vi "Transform And Project.vi"(11 "Core Data":T1={"Screen Dimensions"={"Width"=0, "Height"=0}, "Camera"={"Field Of View"=0.0, "Near Plane"=0.0, "Far Plane"=0.0}, "Transform"={"Position"={"x"=0.0, "y"=0.0, "z"=0.0}, "Rotation"={"x"=0.0, "y"=0.0, "z"=0.0}, "Scale"={"x"=0.0, "y"=0.0, "z"=0.0}}, "Line Colour"=0, "Fill Colour"=0, "Draw Lines"=FALSE, "Projection Matrix"=[], "Update Screen"=FALSE, "Frame Buffer"=refnum, "Objects"=[], "Camera Up"=2.6797385, "Camera Left"=2.6797385, "Camera Rotation"=2.6797385, "Camera Forward"=2.6797385, "Draw Triangles"=FALSE, "Frame Buffer 2"=refnum, "Framebuffer"=FALSE} {"Camera Forward" scale=-10.0..10.0; "Camera Rotation" scale=-90.0..90.0; "Camera Left" scale=-10.0..10.0; "Camera Up" scale=-10.0..10.0}) -> (2 "Delta Time [s]":dbl format="%.3p", 3 "Triangles Sorted":T8[](array[typedef]))   [LabVIEW 2022 SP3]
uses:
  Libraries/3D/Triangle 2D.ctl
  Libraries/3D/Point 2D.ctl
  Core Data.ctl
  Libraries/Raster/Screen Dimensions.ctl
  Libraries/3D/Camera.ctl
  Libraries/3D/Transform.ctl
  Libraries/3D/Vector 3D.ctl
  Libraries/3D/Mesh.ctl
  Libraries/3D/Triangle 3D.ctl
  <vilib>/Utility/High Resolution Relative Seconds.vi
  Libraries/3D/3D.lvlib
  Libraries/Utility/Utility.lvlib
  Libraries/Raster/Raster.lvlib
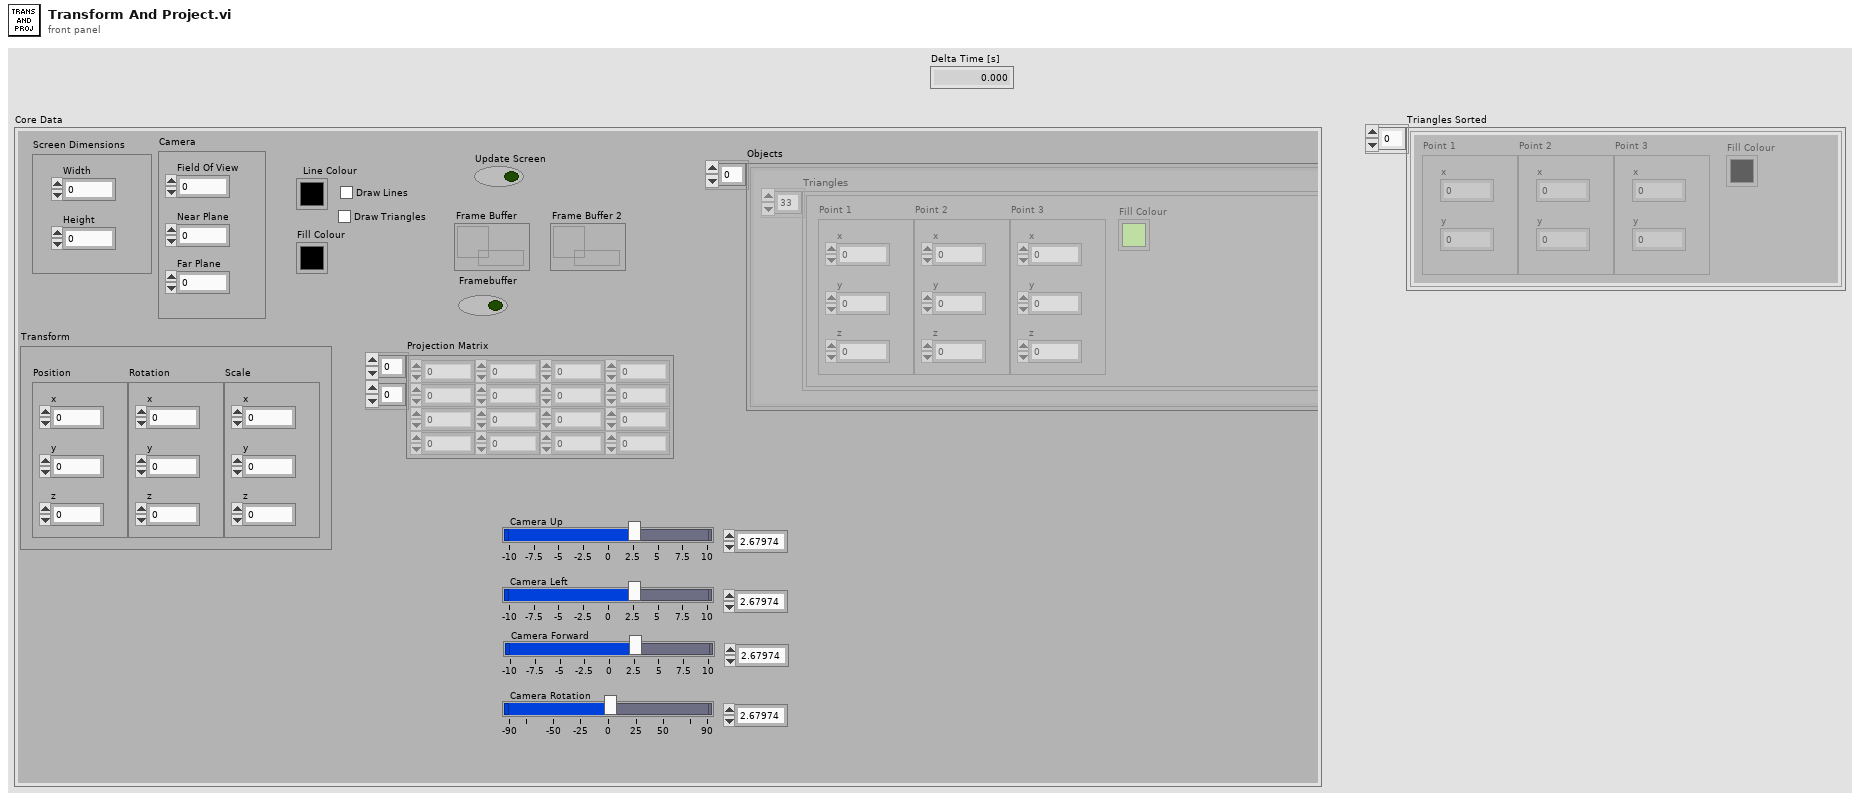
[diagram p1: front panel]
types:
  T1 = typedef "Core Data.ctl" = cluster{"Screen Dimensions":T2, "Camera":T3, "Transform":T4, "Line Colour":u32, "Fill Colour":u32, "Draw Lines":bool, "Projection Matrix":sgl[][], "Update Screen":bool, "Frame Buffer":refnum<data-value>, "Objects":T6[], "Camera Up":sgl, "Camera Left":sgl, "Camera Rotation":sgl, "Camera Forward":sgl, "Draw Triangles":bool, "Frame Buffer 2":refnum<data-value>, "Framebuffer":bool}
  T2 = typedef "Raster.lvlib/Screen Dimensions.ctl" = cluster{"Width":u32, "Height":u32}
  T3 = typedef "3D.lvlib/Camera.ctl" = cluster{"Field Of View":sgl, "Near Plane":sgl, "Far Plane":sgl}
  T4 = typedef "3D.lvlib/Transform.ctl" = cluster{"Position":T5, "Rotation":T5, "Scale":T5}
  T5 = typedef "3D.lvlib/Vector 3D.ctl" = cluster{"x":sgl, "y":sgl, "z":sgl}
  T6 = typedef "3D.lvlib/Mesh.ctl" = cluster{"Triangles":T7[]}
  T7 = typedef "3D.lvlib/Triangle 3D.ctl" = cluster{"Point 1":T5, "Point 2":T5, "Point 3":T5, "Fill Colour":u32}
  T8 = typedef "3D.lvlib/Triangle 2D.ctl" = cluster{"Point 1":T9, "Point 2":T9, "Point 3":T9, "Fill Colour":u32}
  T9 = typedef "3D.lvlib/Point 2D.ctl" = cluster{"x":sgl, "y":sgl}
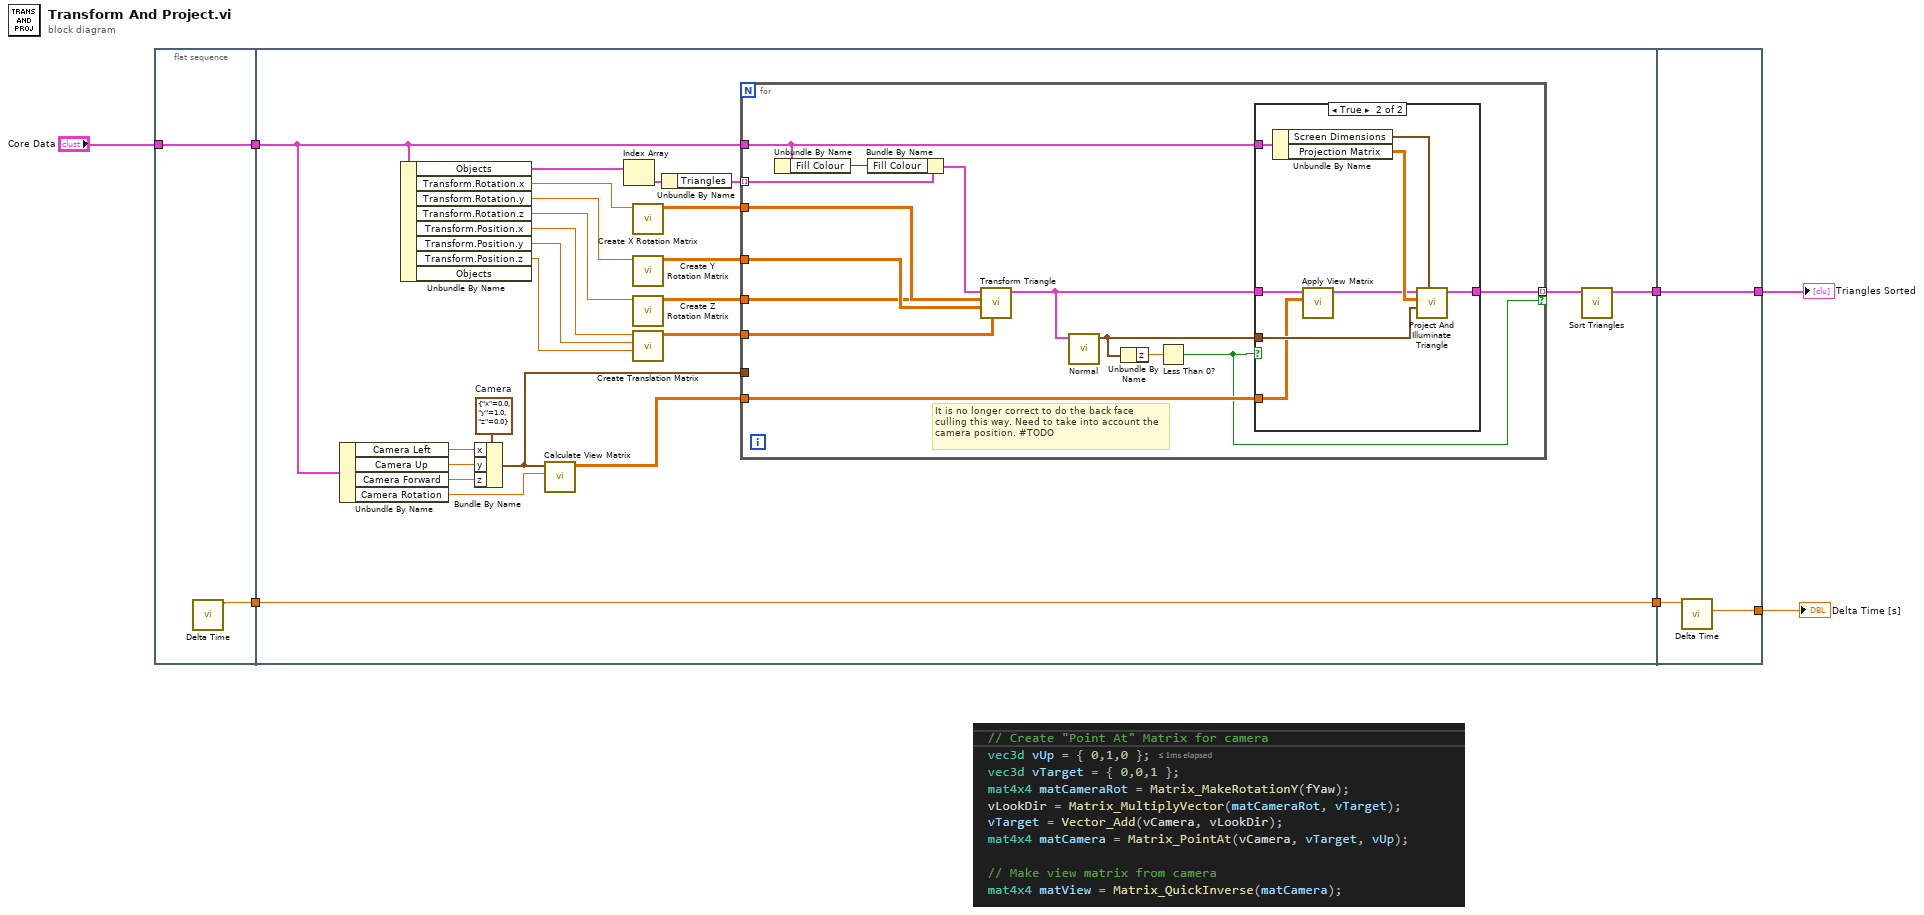
[diagram p0: block diagram]
diagram:
  n1 = flat-sequence {
    tunnel: "Core Data" -> [w9]
    tunnel: [w9] -> w3
    tunnel: [w8] -> w1
    tunnel: [w33] -> w5
    tunnel: w3 -> [w18]
    tunnel: [w10] -> w2
    tunnel: w1 -> [w10]
    tunnel: [w58] -> w7
    tunnel: w5 -> [w58]
    tunnel: [w57] -> w4
    tunnel: w2 -> [w56]
    frame #0 {
      n2 = call "Delta Time.vi"() -> ("Relative Seconds Out"=w8:dbl)  [unwired: 10 in, 1 out]
    }
    frame #1 {
      w17 = T5 {"x"=0.0, "y"=1.0, "z"=0.0}  # Camera
      n3 = Unbundle By Name(w18) -> ("Camera Left"=w12:sgl, "Camera Up"=w13:sgl, "Camera Forward"=w16:sgl, "Camera Rotation"=w14:sgl)
      n4 = Unbundle By Name(w18) -> ("Objects"=w32:T6[], "Transform.Rotation.x"=w26:sgl, "Transform.Rotation.y"=w27:sgl, "Transform.Rotation.z"=w28:sgl, "Transform.Position.x"=w20:sgl, "Transform.Position.y"=w19:sgl, "Transform.Position.z"=w29:sgl)  [unwired: 1 out]
      n5 = Bundle By Name(cluster=w17, "x"=w12, "y"=w13, "z"=w16) -> (w11:T5)
      n6 = call "Calculate View Matrix.vi"("Camera Rotation"=w14, "Camera Position"=w11) -> ("View Matrix"=w15:sgl[][])  [unwired: 9 in]
      n7 = Index Array(array=w32) -> (element=w30:T6)  [unwired: 1 in]
      n8 = call "Create X Rotation Matrix.vi"("Theta (°)"=w26) -> ("Rotation X Matrix"=w23:sgl[][])  [unwired: 10 in]
      n9 = call "Create Y Rotation Matrix.vi"("Theta (°)"=w27) -> ("Rotation Y Matrix"=w24:sgl[][])  [unwired: 10 in]
      n10 = call "Create Z Rotation Matrix.vi"("Theta (°)"=w28) -> ("Rotation Z Matrix"=w22:sgl[][])  [unwired: 10 in]
      n11 = call "Create Translation Matrix.vi"("z"=w29, "y"=w19, "x"=w20) -> ("Translation Matrix"=w25:sgl[][])  [unwired: 8 in]
      n12 = Unbundle By Name(w30) -> ("Triangles"=w31:T7[])
      n13 = for {
        tunnel: w22 -> [w42]
        tunnel: w23 -> [w44]
        tunnel: [w46] -> w21 mode=indexing if=w34
        tunnel: w24 -> [w43]
        tunnel: w25 -> [w41]
        tunnel: w18 -> [w40]
        tunnel: w31 -> [w37] mode=indexing
        tunnel: w15 -> [w36]
        tunnel: w11 -> [_]
        # "It is no longer correct to do the back face culling this way. Need to take into account the camera position. #TODO"
        n14 = Unbundle By Name(w40) -> ("Fill Colour"=w39:u32)
        n15 = Bundle By Name(cluster=w37, "Fill Colour"=w39) -> (w38:T7)
        n16 = call "Transform Triangle.vi"("Translation Matrix"=w41, "Rotation Z Matrix"=w42, "Rotation Y Matrix"=w43, "Rotation X Matrix"=w44, "Triangle in"=w38) -> ("Triangle out"=w35:T7)  [unwired: 6 in]
        n17 = call "Normal.vi"("Triangle"=w35) -> ("Normal"=w45:T5)  [unwired: 10 in]
        n18 = Unbundle By Name(w45) -> ("z"=w47:sgl)
        n19 = Less Than 0?(x=w47) -> (x < 0?=w34:bool)
        n20 = case shown="True" w34 {
          tunnel: [_ w55] -> w46
          tunnel: w45 -> [_ w51]
          tunnel: w40 -> [_ w54]
          tunnel: w35 -> [_ w49]
          tunnel: w36 -> [_ w48]
          frame False {
          }
          frame True {
            n21 = Unbundle By Name(w54) -> ("Screen Dimensions"=w53:T2, "Projection Matrix"=w52:sgl[][])
            n22 = call "Apply View Matrix.vi"("View Matrix"=w48, "Triangle in"=w49) -> ("Triangle"=w50:T7)  [unwired: 9 in]
            n23 = call "Project And Illuminate Triangle.vi"("Screen Dimensions"=w53, "Normal"=w51, "Projection Matrix"=w52, "Triangle in"=w50) -> ("Triangle"=w55:T7)  [unwired: 7 in]
          }
        }
      }
      n24 = call "Sort Triangles.vi"("Triangles"=w21) -> ("Triangles Sorted"=w33:T8[])  [unwired: 10 in]
    }
    frame #2 {
      n25 = call "Delta Time.vi"("Relative Seconds In"=w56) -> ("Delta Time [s]"=w57:dbl)  [unwired: 9 in, 1 out]
    }
  }
  "Triangles Sorted" <- w7
  "Delta Time [s]" <- w4
